vi "2D Chop Integration Bins.vi"(4 "tolerance":dbl=1e-10, 6 "VI ref":cluster{"f(X)":refnum<vi>, "data":variant}, 7 "Formula":T1, 8 "error in (no error)":errorcluster, 9 "Formula/VI ref":bool, 10 "Chop In":bool[](array[boolean]), 11 "Bins In":T2(array[cluster])) -> (0 "error out":errorcluster, 2 "Chop Out":bool[](array[boolean]), 3 "Bins Out":T2(array[cluster]))   [LabVIEW 2018, in "NI_AALPro.lvlib"]
uses:
  NI_AALPro.lvlib
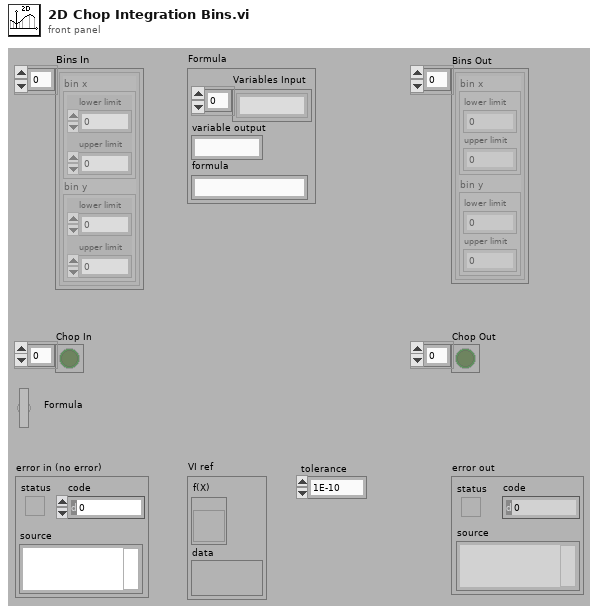
[diagram p1: front panel]
types:
  T1 = cluster{"Variables Input":string[], "variable output":string, "formula":string}
  T2 = cluster{"bin x":cluster{"lower limit":dbl, "upper limit":dbl}, "bin y":cluster{"lower limit":dbl, "upper limit":dbl}}[]
  T3 = cluster{"bin_x":cluster{"lower limit":dbl, "upper limit":dbl}, "bin_y":cluster{"lower limit":dbl, "upper limit":dbl}}[]
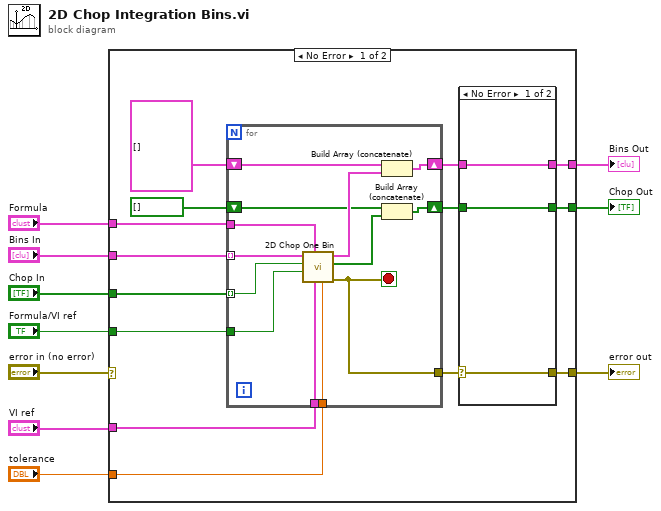
[diagram p0: block diagram]
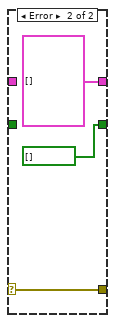
[diagram p2: hidden frame]
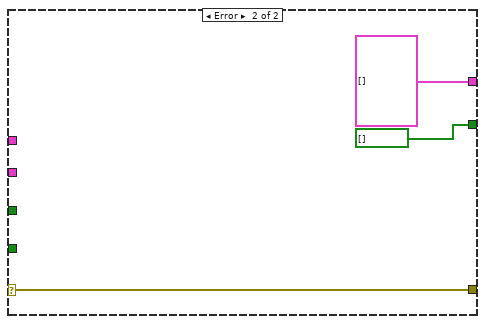
[diagram p3: hidden frame]
diagram:
  n1 = case shown="No Error" "error in (no error)" {
    selector: "error in (no error)" -> [_ w46]
    tunnel: "Bins In" -> [w24 _]
    tunnel: "Formula/VI ref" -> [w23 _]
    tunnel: "VI ref" -> [w22 _]
    tunnel: [w14 T3 []] -> w4
    tunnel: "Chop In" -> [w20 _]
    tunnel: [w12 bool[] []] -> w9
    tunnel: "Formula" -> [w19 _]
    tunnel: [w16 w46] -> w8
    tunnel: "tolerance" -> [w18 _]
    frame No Error {
      n2 = for {
        tunnel: w24 -> [w42] mode=indexing
        tunnel: w23 -> [w35]
        tunnel: w22 -> [w34]
        shift-right: [w38] -> w15
        shift-left: T3 [] -> [w39]
        shift-right: [w43] -> w13
        shift-left: bool[] [] -> [w36]
        tunnel: w20 -> [w41] mode=indexing
        tunnel: w19 -> [w33]
        tunnel: w18 -> [w32]
        tunnel: [w31] -> w11
        stop <- w31 stop-if-true
        n3 = call "2D Chop One Bin.vi"("tolerance"=w32, "VI ref"=w34, "Formula"=w33, "Formula/VI ref"=w35, "chop x?"=w41, "Bins In"=w42) -> ("error out"=w31:errorcluster, "Chop x Out"=w37:bool[], "Bins Out"=w40:T3)  [unwired: 1 in, 2 out]
        n4 = Build Array (concatenate)(w39, w40) -> (w38:T3)
        n5 = Build Array (concatenate)(w36, w37) -> (w43:bool[])
      }
      n6 = case shown="No Error" w11 {
        selector: w11 -> [w27 w28]
        tunnel: [w27 w28] -> w16
        tunnel: w15 -> [w26 _]
        tunnel: [w26 T3 []] -> w14
        tunnel: w13 -> [w25 _]
        tunnel: [w25 bool[] []] -> w12
        frame No Error {
        }
        frame Error {
        }
      }
    }
    frame Error {
    }
  }
  "Chop Out" <- w9
  "error out" <- w8
  "Bins Out" <- w4
